vi "BRig_Host__Loop_Consumer_RunState__closedLoop_parseOutput.vi"(10 "input_pyOut":string) -> ()   [LabVIEW 2014]
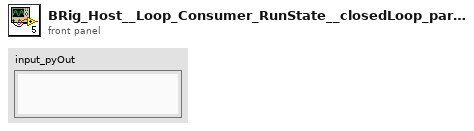
[diagram p1: front panel]
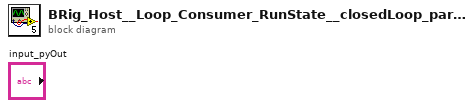
[diagram p0: block diagram]
diagram:
